vi "Teleop.vi"(10 "Match Info":T1={"Autonomous Elapsed Seconds"=0.0, "TeleOp Elapsed Seconds"=0.0, "Disabled Elapsed Seconds"=0.0, "Visited Autonomous"=FALSE, "Visited TeleOp"=FALSE, "Visited Disabled"=FALSE, "Autonomous Settings"={"Autonomous Style"=enum."Independent", "VI Refnum"=refnum}}, 11 "Call Context":T2) -> ()   [LabVIEW 2018]
doc: "This VI is called for each TeleOp packet received from the DS where the robot is not disabled. It is often used to read from the joysticks and update I/O or to update setpoints for timed control loops. It should complete and return within 20 milliseconds or it may miss DS packets."
uses:
  <vilib>/Rock Robotics/WPI/DriverStation/WPI_DriverStationDerivedRobotMode.ctl
  <vilib>/Rock Robotics/WPI/DriverStation/WPI_DriverStationMatch Info.ctl
  <vilib>/Rock Robotics/WPI/Solenoid/WPI_SolenoidValue.ctl
  <vilib>/Rock Robotics/Network Tables/NT Read Boolean.vi
  <vilib>/Rock Robotics/Network Tables/NT Read Number.vi
  <vilib>/Rock Robotics/WPI/ThirdParty/Phoenix-LabVIEW/Motor Controller/Get/CTRE_Phoenix_MotorController_GetSelectedSensorData.vi
  <vilib>/Rock Robotics/WPI/Utilities/WPI_GetSetVariantRefNum.vi
  <vilib>/Rock Robotics/WPI/Solenoid/WPI_SolenoidSetEnum.vi
  Robot Global Data.vi
  FIRST-3958-Controls-Library/NavX/navX Library v2/navX Library v2.lvlib
panel:
  out "element":i16
  in  "set_angle":dbl
  in  "rotation lock":bool
  out "rr_position":i32
  out "rl_position":i32
  out "fr_position":i32
  out "fl_position":i32
  out "Sample Slider 0":dbl(slide) scale=0.0..5.0
  out "Sample Boolean 1":bool
  out "Sample Boolean 0":bool
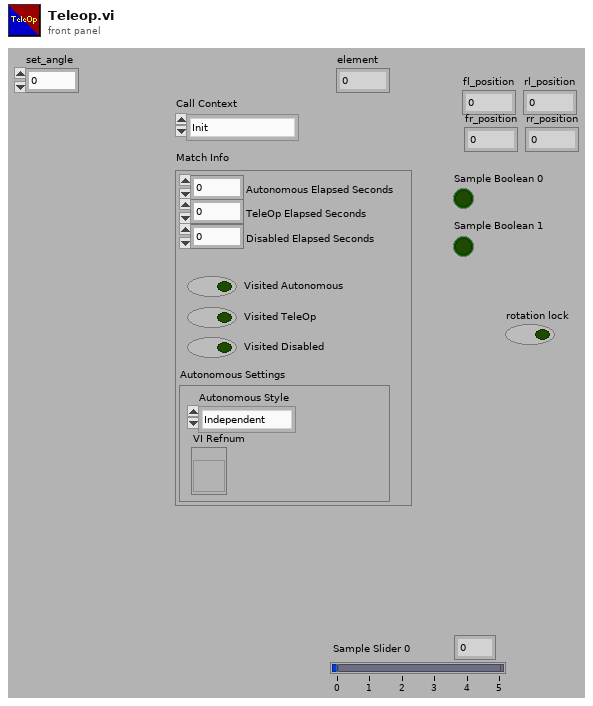
[diagram p1: front panel]
types:
  T1 = typedef "WPI_DriverStationMatch Info.ctl" = cluster{"Autonomous Elapsed Seconds":dbl, "TeleOp Elapsed Seconds":dbl, "Disabled Elapsed Seconds":dbl, "Visited Autonomous":bool, "Visited TeleOp":bool, "Visited Disabled":bool, "Autonomous Settings":cluster{"Autonomous Style":enum16{"Iterative", "Independent"}, "VI Refnum":refnum<vi>}}
  T2 = typedef "WPI_DriverStationDerivedRobotMode.ctl" = enum16{"Init", "Execute", "Stop"}
  T3 = typedef "WPI_SolenoidValue.ctl" = enum16{"Off", "On", "Forward", "Reverse"}
  T4 = typedef "WPI_JoystickDevRef.ctl" = cluster{"Device":T5}
  T5 = typedef "WPI_JoystickDeviceEnum.ctl" = enum16{"USB 0", "USB 1", "USB 2", "USB 3", "USB 4", "USB 5"}
  T6 = typedef "navX Library v2.lvlib/Z900_navX_DeviceTypeDef.ctl" = cluster{"Interface":cluster{"Protocol":T7, "Update Rate (4Hz-100Hz)":u8, "navX Open TypeDef":variant}, "Notify Packet":refnum<notifier>, "Loop VI Refnum":refnum<vi>, "Ready to Close Occurrence Refnum":refnum<k4>}
  T7 = typedef "navX Library v2.lvlib/Z900_navX_ProtocolTypeDef.ctl" = enum16{"SERIAL", "I2C", "SPI"}
  T8 = typedef "WPI_MotorControlDeviceRef.ctl" = cluster{"DeviceStatus":errorcluster, "Type":T9, "PWM":cluster{"PWM Channel":T10, "DeadBand":T11}, "CAN":cluster{"Device Number":u8, "SetOutput VI Ref":variant, "GetOutput VI Ref":variant, "Enable VI Ref":variant, "Disable VI Ref":variant, "Data":variant}, "Invert":bool, "DIO PWM":cluster{"PWM \"Enable\" Channel":T10, "DIOChannel":T12, "PWM Rate":dbl}}
  T9 = typedef "WPI_MotorControlType.ctl" = enum16{"PWM", "CAN", "DIO PWM"}
  T10 = typedef "FPGA_DIOPWMChannel.ctl" = enum8{"PWM 0", "PWM 1", "PWM 2", "PWM 3", "PWM 4", "PWM 5", "PWM 6", "PWM 7", "PWM 8", "PWM 9", "PWM MXP 0", "PWM MXP 1", "PWM MXP 2", "PWM MXP 3", "PWM MXP 4", "PWM MXP 5", "PWM MXP 6", "PWM MXP 7", "PWM MXP 8", "PWM MXP 9", "Invalid"}
  T11 = typedef "WPI_PWMDeadband.ctl" = cluster{"Name":string, "maxPositivePwm":i32, "minPositivePwm":i32, "centerPwm":i32, "maxNegativePwm":i32, "minNegativePwm":i32, "angularRange":u16}
  T12 = typedef "FPGA_DIOChannel.ctl" = enum8{"DIO 0", "DIO 1", "DIO 2", "DIO 3", "DIO 4", "DIO 5", "DIO 6", "DIO 7", "DIO 8", "DIO 9", "DIO MXP 0", "DIO MXP 1", "DIO MXP 2", "DIO MXP 3", "DIO MXP 4", "DIO MXP 5", "DIO MXP 6", "DIO MXP 7", "DIO MXP 8", "DIO MXP 9", "DIO MXP 10", "DIO MXP 11", "DIO MXP 12", "DIO MXP 13", "DIO MXP 14", "DIO MXP 15", "SPI Port CS1", "SPI Port CS2", "SPI Port CS3", "SPI Port MISO", "SPI Port MOSI", "Invalid"}
  T13 = cluster{"Yaw":dbl, "Roll":dbl, "Pitch":dbl, "Heading":dbl, "Fused Heading":dbl}
  T14 = typedef "WPI_SolenoidDevRef.ctl" = cluster{"DevStatus":errorcluster, "Pneumatics Control Module":u8, "Forward Solenoid Channel":T15, "Reverse Solenoid Channel":T15}
  T15 = typedef "WPI_SolenoidChannel.ctl" = enum8{"Solenoid 0", "Solenoid 1", "Solenoid 2", "Solenoid 3", "Solenoid 4", "Solenoid 5", "Solenoid 6", "Solenoid 7", "Invalid"}
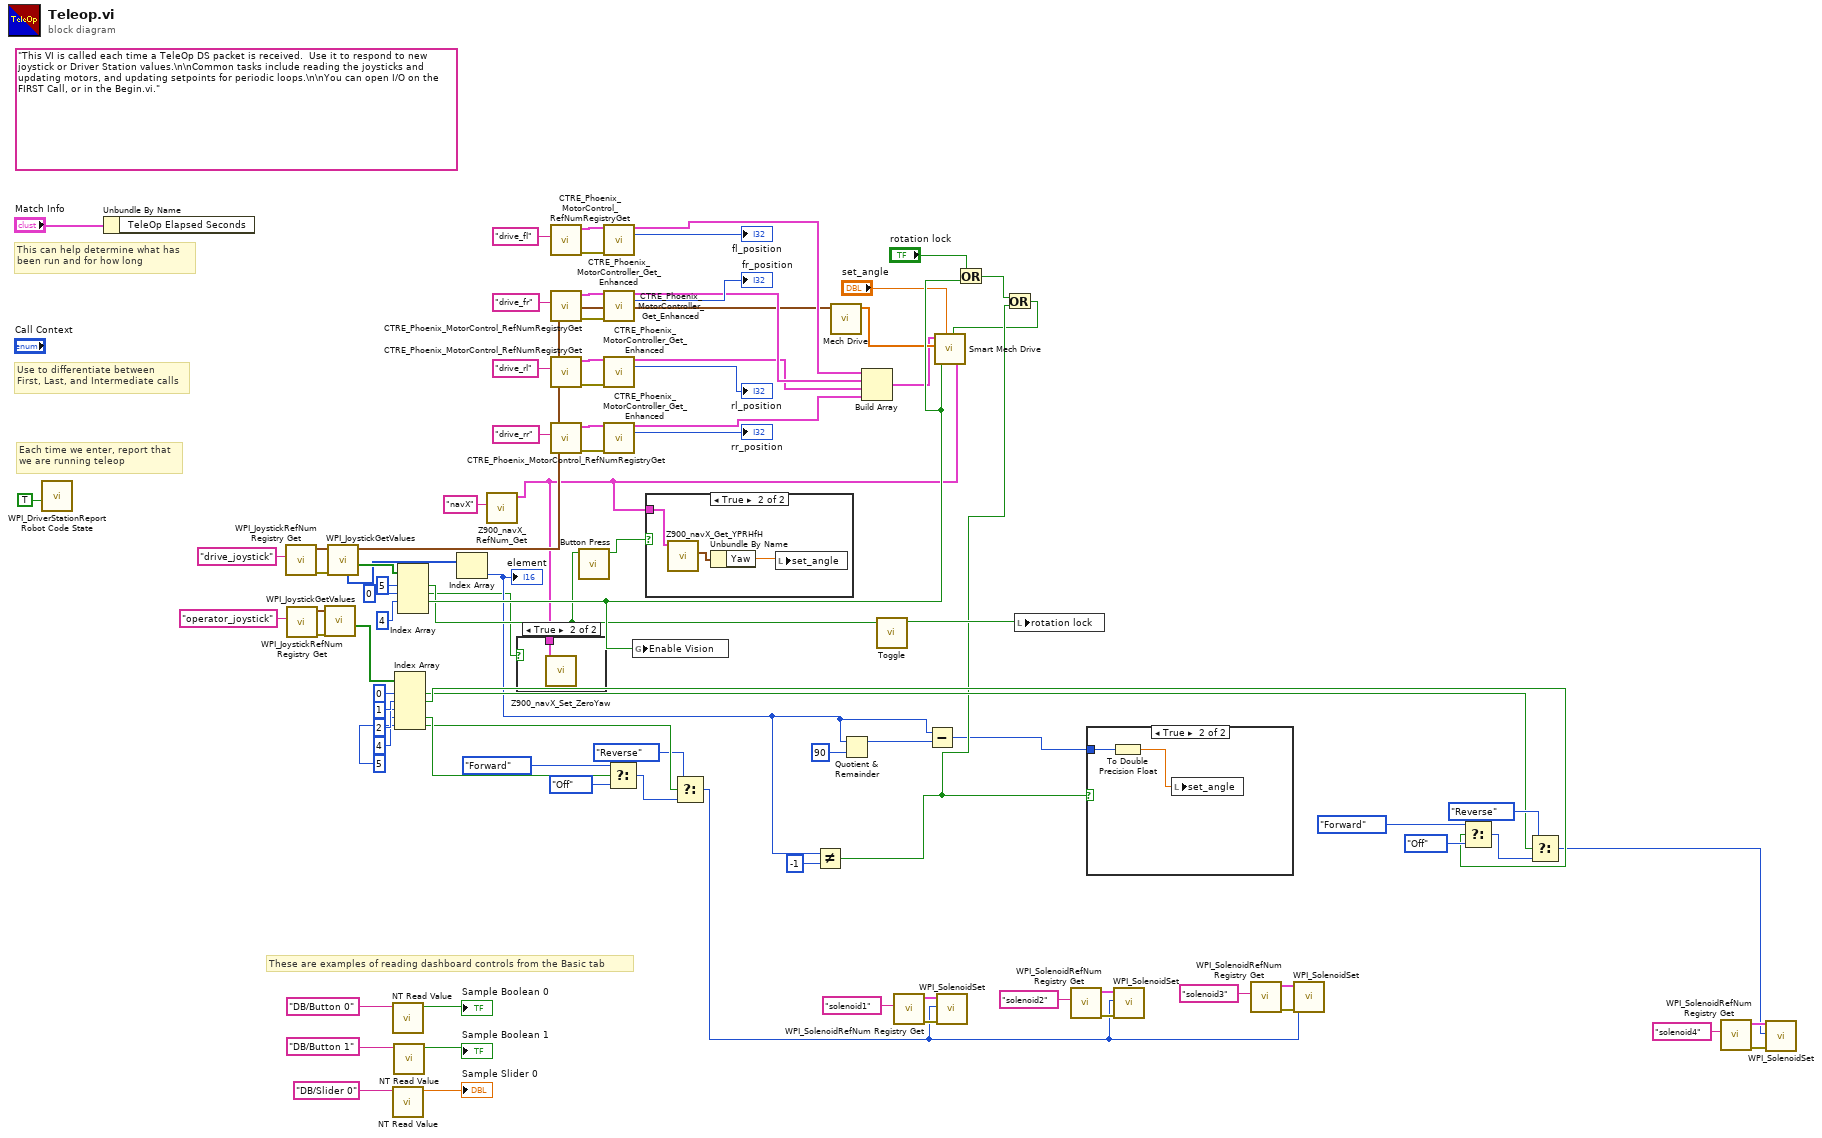
[diagram p0: block diagram]
diagram:
  (unwired) "This VI is called each time a TeleOp DS packet is received.  Use it to respond to new joystick or Driver Station values.\n\nCommon tasks include reading the joysticks and updating motors, and updating setpoints for periodic loops.\n\nYou can open I/O on the FIRST Call, or in the Begin.vi."
  # "These are examples of reading dashboard controls from the Basic tab"
  # "Each time we enter, report that\nwe are running teleop"
  # "Use to differentiate between\nFirst, Last, and Intermediate calls"
  # "This can help determine what has\nbeen run and for how long"
  n1 = call <vilib>:"WPI_DriverStationReport Robot Code State.vi"("TeleOp"=TRUE ("Autonomous")) -> ()  [unwired: 10 in, 1 out]
  n2 = Unbundle By Name("Match Info") -> ()  [unwired: 1 out]
  n3 = call <vilib>:"WPI_JoystickRefNum Registry Get.vi"("refnum name"="drive_joystick") -> ("error out"=w66:errorcluster, "JoystickDevRef"=w65:T4)  [unwired: 9 in]
  n4 = call <vilib>:"WPI_JoystickRefNum Registry Get.vi"("refnum name"="operator_joystick") -> ("error out"=w55:errorcluster, "JoystickDevRef"=w54:T4)  [unwired: 9 in]
  n5 = call <vilib>:"WPI_JoystickGetValues.vi"("error in (no error)"=w55, "JoystickDevRef"=w54) -> ("Buttons"=w52:bool[])  [unwired: 5 in, 4 out]
  n6 = call <vilib>:"WPI_JoystickGetValues.vi"("error in (no error)"=w66, "JoystickDevRef"=w65) -> ("Buttons"=w51:bool[], "JoystickDevRef"=w11:T4, "POVs"=w13:i16[])  [unwired: 5 in, 2 out]
  n7 = call-poly <vilib>:"NT Read Value.vi"("Name"="DB/Button 0" ("refnum name")) -> ("Boolean"=→"Sample Boolean 0":bool)  [unwired: 9 in, 1 out]
  n8 = call-poly <vilib>:"NT Read Value.vi"("Name"="DB/Slider 0" ("refnum name")) -> ("Numeric"=→"Sample Slider 0":dbl)  [unwired: 9 in, 1 out]
  n9 = call-poly <vilib>:"NT Read Value.vi"("Name"="DB/Button 1" ("refnum name")) -> ("Boolean"=→"Sample Boolean 1":bool)  [unwired: 9 in, 1 out]
  n10 = Index Array(array=w52, index #1=0 ("index"), index #2=1 ("index"), index #3=2 ("index"), index #4=4 ("index"), index #5=5 ("index")) -> (element #1=w26:bool, element #2=w27:bool, element #4=w38:bool, element #5=w37:bool)  [unwired: 1 out]
  n11 = Index Array(array=w51, index #1=5 ("index"), index #2=0 ("index"), index #3=4 ("index")) -> (element #1=w14:bool, element #2=w3:bool, element #3=w23:bool)  [unwired: 1 in, 1 out]
  n12 = Index Array(array=w13) -> (element=w9:i16)  [unwired: 1 in]
  "element" <- w9
  n13 = call "Z900_navX_RefNum_Get.vi"("refnum name"="navX") -> ("navX Device"=w2:T6)  [unwired: 9 in, 1 out]
  n14 = case shown="True" w3 {
    tunnel: w2 -> [_ w92]
    frame False {
    }
    frame True {
      n15 = call "Z900_navX_Set_ZeroYaw.vi"("navX Device"=w92) -> ()  [unwired: 9 in, 2 out]
    }
  }
  n16 = call <vilib>:"CTRE_Phoenix_MotorControl_RefNumRegistryGet.vi"("refnum name"="drive_fl") -> ("error out"=w78:errorcluster, "PhoenixMotorControlDevRef"=w79:T8)  [unwired: 9 in]
  n17 = call <vilib>:"CTRE_Phoenix_MotorControl_RefNumRegistryGet.vi"("refnum name"="drive_fr") -> ("error out"=w76:errorcluster, "PhoenixMotorControlDevRef"=w77:T8)  [unwired: 9 in]
  n18 = call <vilib>:"CTRE_Phoenix_MotorControl_RefNumRegistryGet.vi"("refnum name"="drive_rl") -> ("error out"=w74:errorcluster, "PhoenixMotorControlDevRef"=w75:T8)  [unwired: 9 in]
  n19 = call <vilib>:"CTRE_Phoenix_MotorControl_RefNumRegistryGet.vi"("refnum name"="drive_rr") -> ("error out"=w72:errorcluster, "PhoenixMotorControlDevRef"=w73:T8)  [unwired: 9 in]
  n20 = call "Button Press.vi"("Button In"=w14) -> ("Button Pressed?"=w15:bool)  [unwired: 10 in]
  n21 = call-poly <vilib>:"CTRE_Phoenix_MotorController_Get_Enhanced.vi"("PhoenixMotorControlDevRef"=w79, "error in"=w78) -> ("PhoenixMotorControlDevRef"=w21:T8, "Position (Raw Sensor Units)"=→"fl_position":i32)  [unwired: 10 in, 2 out]
  n22 = call-poly <vilib>:"CTRE_Phoenix_MotorController_Get_Enhanced.vi"("PhoenixMotorControlDevRef"=w77, "error in"=w76) -> ("PhoenixMotorControlDevRef"=w20:T8, "Position (Raw Sensor Units)"=→"fr_position":i32)  [unwired: 10 in, 2 out]
  n23 = call-poly <vilib>:"CTRE_Phoenix_MotorController_Get_Enhanced.vi"("PhoenixMotorControlDevRef"=w75, "error in"=w74) -> ("PhoenixMotorControlDevRef"=w19:T8, "Position (Raw Sensor Units)"=→"rl_position":i32)  [unwired: 10 in, 2 out]
  n24 = call-poly <vilib>:"CTRE_Phoenix_MotorController_Get_Enhanced.vi"("PhoenixMotorControlDevRef"=w73, "error in"=w72) -> ("PhoenixMotorControlDevRef"=w18:T8, "Position (Raw Sensor Units)"=→"rr_position":i32)  [unwired: 10 in, 2 out]
  n25 = Select(t=WPI_SolenoidValue."Forward", s=w38, f=WPI_SolenoidValue."Off") -> (s? t:f=w34:T3)
  n26 = global write "Robot Global Data.vi" "Enable Vision"(w23) -> ()
  n27 = case shown="True" w15 {
    tunnel: w2 -> [_ w95]
    frame False {
    }
    frame True {
      n28 = call "Z900_navX_Get_YPRHfH.vi"("navX Device"=w95) -> ("YRPHfH"=w94:T13)  [unwired: 7 in, 3 out]
      n29 = Unbundle By Name(w94) -> ("Yaw"=w93:dbl)
      n30 = local write "set_angle"(w93) -> ()
    }
  }
  n31 = Select(t=WPI_SolenoidValue."Reverse", s=w37, f=w34) -> (s? t:f=w32:T3)
  n32 = Not Equal?(x=w9, y=i16 -1) -> (x != y?=w6:bool)
  n33 = call "Mech Drive.vi"("JoystickDevRef"=w11) -> ("motor values"=w22:dbl[])  [unwired: 10 in]
  n34 = Quotient & Remainder(x=w9, y=i16 90) -> (x-y*floor(x/y)=w10:i16)  [unwired: 1 out]
  n35 = Build Array(w21, w20, w19, w18) -> (w17:T8[])
  n36 = call "Toggle.vi"("Button Input"=w14) -> ("Toggle Output"=w56:bool)  [unwired: 9 in, 1 out]
  n37 = call <vilib>:"WPI_SolenoidRefNum Registry Get.vi"("refnum name"="solenoid1") -> ("error out"=w42:errorcluster, "SolenoidDevRef"=w43:T14)  [unwired: 9 in]
  n38 = Subtract(x=w9, y=w10) -> (x-y=w1:i16)
  n39 = call-poly <vilib>:"WPI_SolenoidSet.vi"("error in (no error)"=w42, "Value"=w32, "SolenoidDevRef"=w43) -> ()  [unwired: 7 in, 2 out]
  n40 = Or(x="rotation lock", y=w23) -> (x .or. y?=w7:bool)
  n41 = Or(x=w7, y=w6) -> (x .or. y?=w5:bool)
  n42 = call "Smart Mech Drive.vi"("navX Device"=w2, "rotation lock"=w5, "align"=w23, "set_angle"="set_angle", "motor values"=w22, "appended array"=w17) -> ()  [unwired: 2 in, 4 out]
  n43 = local write "rotation lock"(w56) -> ()
  n44 = call <vilib>:"WPI_SolenoidRefNum Registry Get.vi"("refnum name"="solenoid2") -> ("error out"=w44:errorcluster, "SolenoidDevRef"=w45:T14)  [unwired: 9 in]
  n45 = case shown="True" w6 {
    tunnel: w1 -> [_ w96]
    frame False {
    }
    frame True {
      n46 = To Double Precision Float(number=w96) -> (double precision float=w97:dbl)
      n47 = local write "set_angle"(w97) -> ()
    }
  }
  n48 = call-poly <vilib>:"WPI_SolenoidSet.vi"("error in (no error)"=w44, "Value"=w32, "SolenoidDevRef"=w45) -> ()  [unwired: 7 in, 2 out]
  n49 = call <vilib>:"WPI_SolenoidRefNum Registry Get.vi"("refnum name"="solenoid3") -> ("error out"=w46:errorcluster, "SolenoidDevRef"=w47:T14)  [unwired: 9 in]
  n50 = call-poly <vilib>:"WPI_SolenoidSet.vi"("error in (no error)"=w46, "Value"=w32, "SolenoidDevRef"=w47) -> ()  [unwired: 7 in, 2 out]
  n51 = Select(t=WPI_SolenoidValue."Forward", s=w27, f=WPI_SolenoidValue."Off") -> (s? t:f=w29:T3)
  n52 = Select(t=WPI_SolenoidValue."Reverse", s=w26, f=w29) -> (s? t:f=w25:T3)
  n53 = call <vilib>:"WPI_SolenoidRefNum Registry Get.vi"("refnum name"="solenoid4") -> ("error out"=w61:errorcluster, "SolenoidDevRef"=w60:T14)  [unwired: 9 in]
  n54 = call-poly <vilib>:"WPI_SolenoidSet.vi"("error in (no error)"=w61, "Value"=w25, "SolenoidDevRef"=w60) -> ()  [unwired: 7 in, 2 out]
